vi "PADMINI_AUTO_CYCLE TIME 100.vi"(7 "Enum":enum16{"Read", "Write"}(ring), 8 "error in (no error)":errorcluster, 11 "Time of Day result array in":timestamp[](array[timestamp])=[timestamp(0 s since 1904-01-01), timestamp(27000 s since 1904-01-01)] format="%<%.3X>T") -> (0 "error out":errorcluster, 3 "Time of Day result array":timestamp[](array[timestamp])=[timestamp(0 s since 1904-01-01), timestamp(27000 s since 1904-01-01)] format="%<%.3X>T")   [LabVIEW 2017]
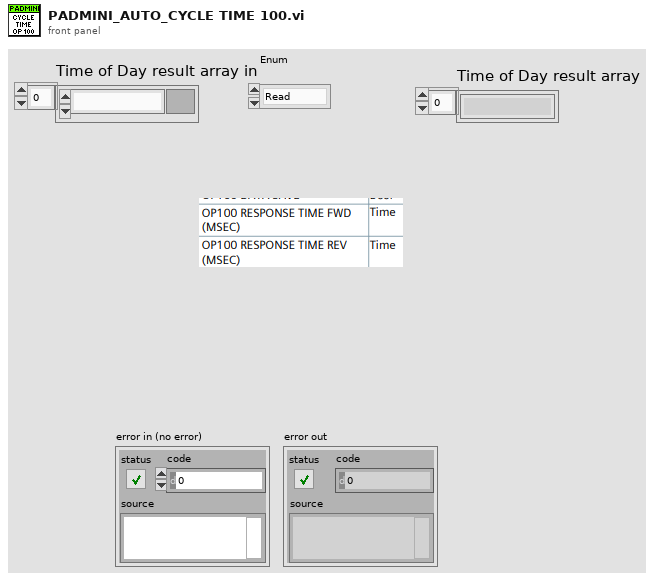
[diagram p1: front panel]
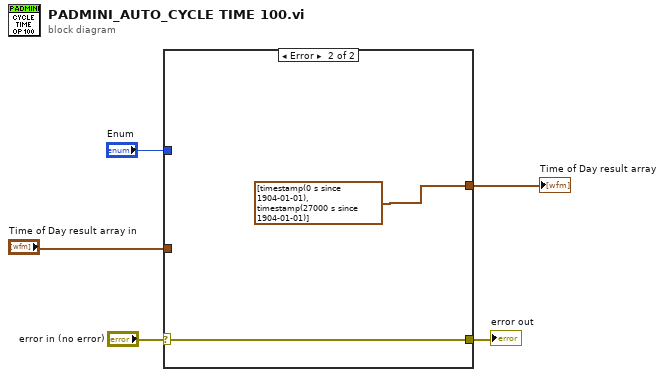
[diagram p0: block diagram]
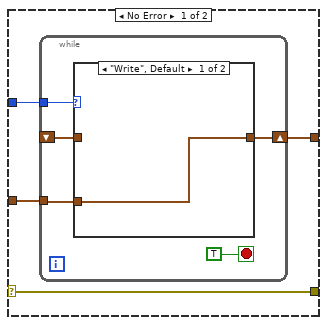
[diagram p2: hidden frame]
diagram:
  n1 = case shown="Error" "error in (no error)" {
    selector: "error in (no error)" -> [w6 w18]
    tunnel: "Enum" -> [w9 _]
    tunnel: "Time of Day result array in" -> [w8 _]
    tunnel: [w7 timestamp[] [timestamp(0 s since 1904-01-01), timestamp(27000 s since 1904-01-01)] ("Time of Day result array")] -> w2
    tunnel: [w6 w18] -> w3
    frame No Error {
      n2 = while {
        tunnel: w9 -> [w14]
        shift-right: [w12] -> w7
        shift-left: _ -> [w11]
        tunnel: w8 -> [w13]
        stop <- TRUE stop-if-true
        n3 = case shown="\"Write\", Default" w14 {
          tunnel: [w15 w16] -> w12
          tunnel: w13 -> [w15 _]
          tunnel: w11 -> [_ w16]
          frame "Write", Default {
          }
          frame "Read" {
          }
        }
      }
    }
    frame Error {
    }
  }
  "error out" <- w3
  "Time of Day result array" <- w2
